vi "ReportWriteFileHeader.vi"(4 "Results":string[][](array[string]), 8 "error in":errorcluster, 10 "Report File Header":T2, 11 "Report File Path":path) -> (0 "error out":errorcluster, 2 "file offset":i32, 3 "Report File Path out":path)   [LabVIEW 2022 SP3]
doc: "This VI store the header information in to the result file. \nAs input the string cluster is necessary to fill out all information"
uses:
  <vilib>/Utility/file.llb/Write Delimited Spreadsheet (string).vi
panel:
  out "VI_State":T1(ring)
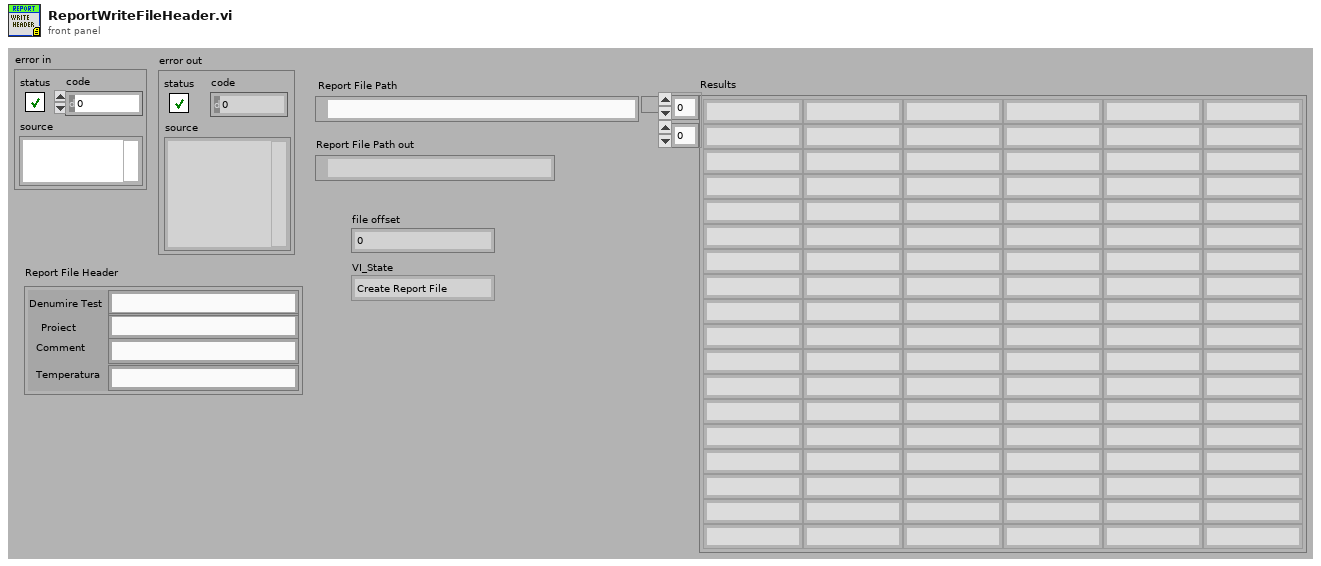
[diagram p1: front panel]
types:
  T1 = enum8{"Create Report File", "Open Report File", "Convert Header Data", "Write Data to File", "Close Report File"}
  T2 = cluster{"Denumire Test":string, "Proiect":string, "Comment":string, "Test prog name":string, "Test prog version":string, "Temperatura":string}
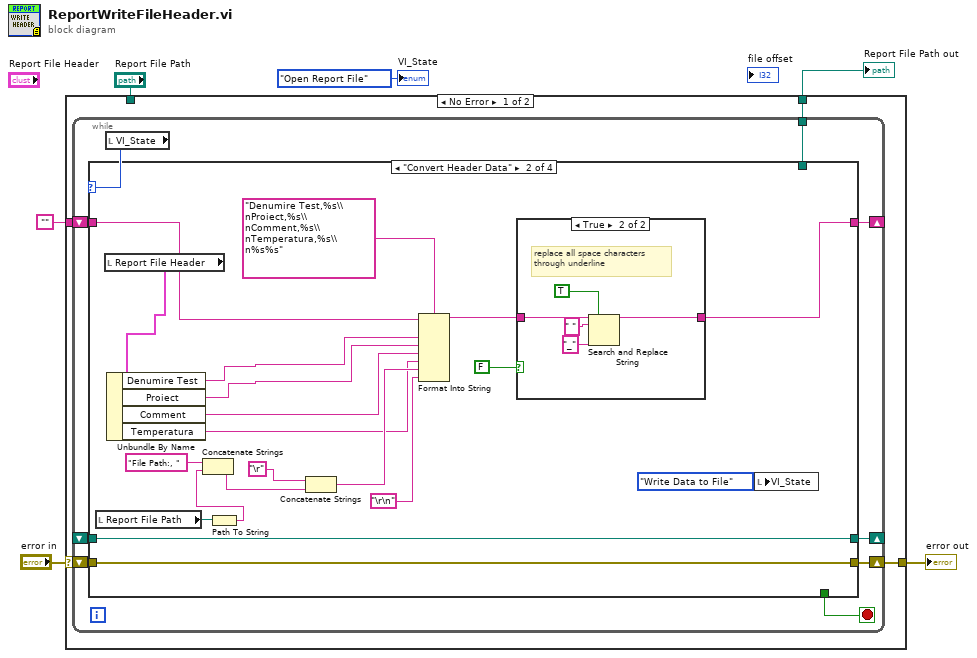
[diagram p0: block diagram]
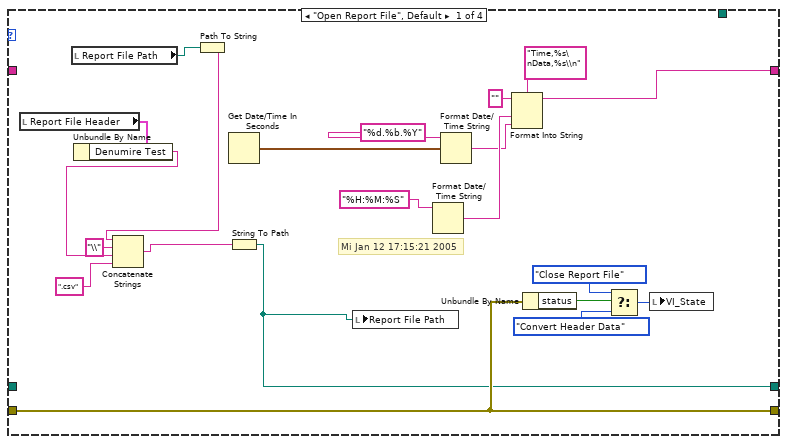
[diagram p2: hidden frame]
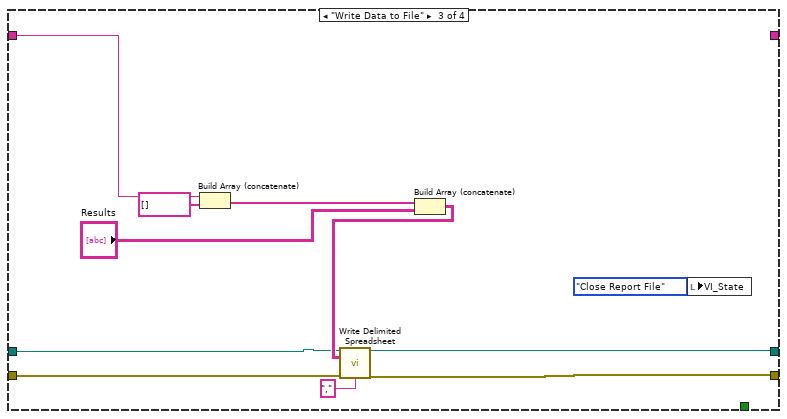
[diagram p4: hidden frame]
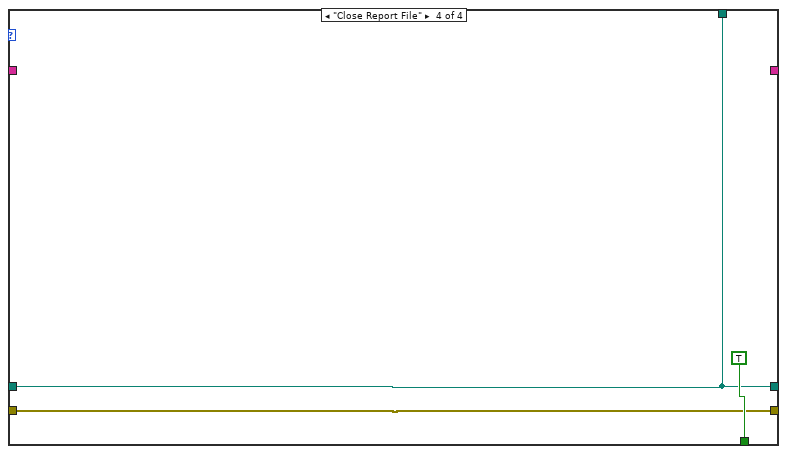
[diagram p5: hidden frame]
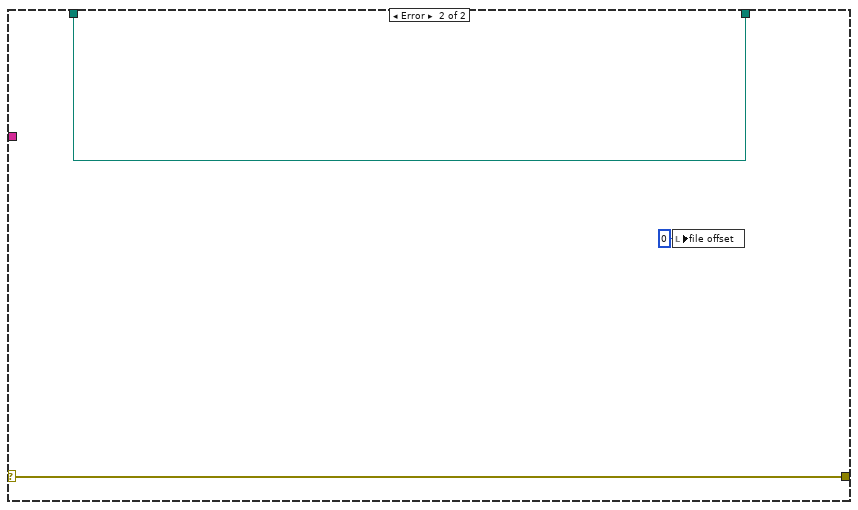
[diagram p6: hidden frame]
diagram:
  n1 = case shown="No Error" "error in" {
    selector: "error in" -> [w10 w83]
    tunnel: [w9 w83] -> w5
    tunnel: [w8 w82] -> w4
    tunnel: "Report File Path" -> [_ w82]
    tunnel: "" -> [w7 _]
    frame No Error {
      n2 = while {
        tunnel: [w12] -> w8
        shift-right: [w15] -> _
        shift-left: w7 -> [w11]
        shift-right: [w14] -> _
        shift-left: _ -> [w13]
        shift-right: [w17] -> w9
        shift-left: w10 -> [w18]
        stop <- w16 stop-if-true
        n3 = local read "VI_State"() -> (w19:T1)
        n4 = case shown="\"Convert Header Data\"" w19 {
          tunnel: w18 -> [w28 w60 w68 w79]
          tunnel: [w28 w60 w71 w79] -> w17
          tunnel: [_ _ _ TRUE] -> w16
          tunnel: [w37 w55 _ _] -> w15
          tunnel: [w23 w59 w70 w78] -> w14
          tunnel: w13 -> [_ w59 w69 w78]
          tunnel: [_ _ _ w78] -> w12
          tunnel: w11 -> [_ w58 w76 _]
          frame "Open Report File", Default {
            # "Mi Jan 12 17:15:21 2005"
            n5 = local read "Report File Header"() -> (w27:T2)
            n6 = local read "Report File Path"() -> (w25:path)
            n7 = Unbundle By Name(w27) -> ("Denumire Test"=w21:string)
            n8 = Path To String(path=w25) -> (string=w24:string)
            n9 = Concatenate Strings(w24, "\\" ("string"), w21, ".csv" ("string")) -> (w26:string)
            n10 = Get Date/Time In Seconds() -> (seconds since 1Jan1904=w40:timestamp)
            n11 = String To Path(string=w26) -> (path=w23:path)
            n12 = local write "Report File Path"(w23) -> ()
            n13 = Format Date/Time String(time format string (%c)="%H:%M:%S") -> (date/time string=w31:string)  [unwired: 2 in]
            n14 = Format Date/Time String(time format string (%c)="%d.%b.%Y", seconds (now)=w40) -> (date/time string=w30:string)  [unwired: 1 in]
            n15 = Format Into String(format string="Time,%s\nData,%s\\n", initial string="", w31, w30) -> (resulting string=w37:string)  [unwired: 1 in, 1 out]
            n16 = Unbundle By Name(w28) -> ("status"=w36:bool)
            n17 = Select(t=T1."Close Report File" ("VI_State"), s=w36, f=T1."Convert Header Data" ("VI_State")) -> (s? t:f=w33:T1)
            n18 = local write "VI_State"(w33) -> ()
          }
          frame "Convert Header Data" {
            n19 = local read "Report File Path"() -> (w51:path)
            n20 = local read "Report File Header"() -> (w47:T2)
            n21 = Unbundle By Name(w47) -> ("Denumire Test"=w42:string, "Proiect"=w46:string, "Comment"=w44:string, "Temperatura"=w43:string)
            n22 = Path To String(path=w51) -> (string=w41:string)
            n23 = Concatenate Strings("File Path:, " ("string"), w41) -> (w50:string)
            n24 = Concatenate Strings("\r", w50) -> (w49:string)
            n25 = Format Into String(format string="Denumire Test,%s\\nProiect,%s\\nComment,%s\\nTemperatura,%s\\n%s%s", initial string=w58, w42, w46, w44, w43, w49, "\r\n") -> (resulting string=w56:string)  [unwired: 1 in, 1 out]
            n26 = case shown="True" FALSE {
              tunnel: w56 -> [w61 w65]
              tunnel: [w61 w62] -> w55
              frame False {
              }
              frame True {
                # "replace all space characters through underline"
                n27 = Search and Replace String(replace all?=TRUE ("replace all? (F)"), input string=w65, search string=" ", replace string="_" ("replace string (\"\")")) -> (result string=w62:string)  [unwired: 4 in, 3 out]
              }
            }
            n28 = local write "VI_State"(T1."Write Data to File" ("VI_State")) -> ()
          }
          frame "Write Data to File" {
            n29 = Build Array (concatenate)(w76, string[] [] ("array")) -> (w74:string[])
            n30 = Build Array (concatenate)(w74, "Results") -> (w72:string[][])
            n31 = call-poly <vilib>:"Write Delimited Spreadsheet.vi"("file path (dialog if empty)"=w69, "2D data"=w72, "error in (no error)"=w68, "delimiter (\\t)"="," ("delimiter (\\t)")) -> ("new file path (Not A Path if cancelled)"=w70:path, "error out"=w71:errorcluster)  [unwired: 10 in]
            n32 = local write "VI_State"(T1."Close Report File" ("VI_State")) -> ()
          }
          frame "Close Report File" {
          }
        }
      }
    }
    frame Error {
      n33 = local write "file offset"(0 ("file offset")) -> ()
    }
  }
  "error out" <- w5
  "Report File Path out" <- w4
  "VI_State" <- T1."Open Report File" ("VI_State")
